vi "Columns.vi"() -> (2 "Columns":T1)   [LabVIEW 2020, in "tests.lvlib" / "LiveDemo.lvclass"]
uses:
  LiveDemo.lvclass
  Columns.ctl
  <vilib>/IlluminatedG/IG Conditum Base/Conditum/Columns/Boolean/Boolean.lvclass
  <vilib>/IlluminatedG/IG Conditum Base/Conditum/Columns/Double/Double.lvclass
  <vilib>/IlluminatedG/IG Conditum Base/Conditum/Columns/String/String.lvclass
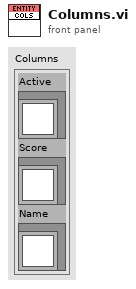
[diagram p1: front panel]
types:
  T1 = typedef "tests.lvlib/LiveDemo.lvclass/Columns.ctl" = cluster{"Active":refnum<class "Boolean.lvclass">, "Score":refnum<class "Double.lvclass">, "Name":refnum<class "String.lvclass">}
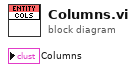
[diagram p0: block diagram]
diagram:
